vi "initialise.vi"(8 "error in (no error)":errorcluster, 11 "Stimulator090724 in":refnum<class "StimulatorDL090727Writer.lvclass">) -> (0 "error out":errorcluster, 3 "Stimulator090724 out":refnum<class "StimulatorDL090727Writer.lvclass">)   [LabVIEW 2010, in "StimulatorDL090727Writer.lvclass"]
doc: "The dynamic dispatch-version of this VI initalises the plug-in object by allocating and initalising any dynamic resources need."
uses:
  StimulatorDL090727Writer.lvclass
  common/enumerations/functional_global_action_enum.ctl
  StimulatorDL090727Writer.lvclass/StimulatorDL090727Writer.ctl
  SignalWriter/GenericSignalWriter/GenericSignalWriter/GenericSignalWriter.lvclass
  StimulatorDL090724Scaffold/StimulatorDL090724Scaffold/Stimulator090724Scaffold.lvclass
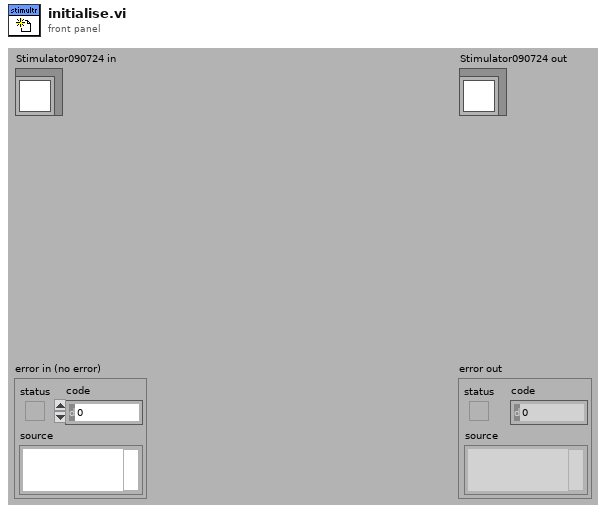
[diagram p1: front panel]
types:
  T1 = typedef "functional_global_action_enum.ctl" = enum16{"get", "set", "reset"}
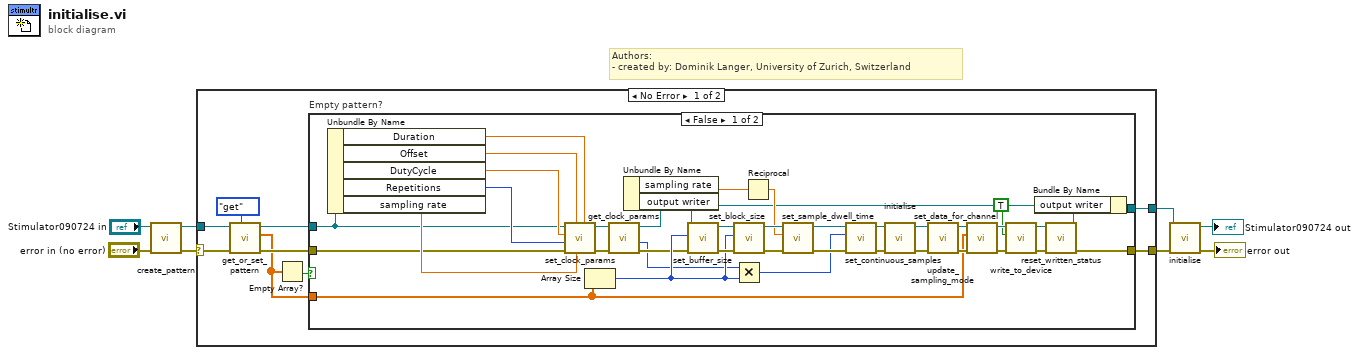
[diagram p0: block diagram]
diagram:
  # "Authors: \n- created by: Dominik Langer, University of Zurich, Switzerland"
  n1 = call-dynamic "create_pattern.vi"("error in (no error)"="error in (no error)", "StimulatorDL090727DAQmx in"="Stimulator090724 in") -> ("error out"=w4:errorcluster, "StimulatorDL090727DAQmx out"=w3:refnum<class "StimulatorDL090727Writer.lvclass">)  [unwired: 8 out]
  n2 = case shown="No Error" w4 {
    selector: w4 -> [w14 w58]
    tunnel: w3 -> [w13 w59]
    tunnel: [w16 w58] -> w2
    tunnel: [w15 w59] -> w1
    frame No Error {
      n3 = call-dynamic "get_or_set_pattern.vi"("action"=functional_global_action_enum."get", "error in (no error)"=w14, "Stimulator090724 in"=w13) -> ("error out"=w12:errorcluster, "samples out"=w10:dbl[], "Stimulator090724 out"=w11:refnum<class "StimulatorDL090727Writer.lvclass">)  [unwired: 1 in, 5 out]
      n4 = Empty Array?(array=w10) -> (empty?=w9:bool)
      n5 = case "Empty pattern?" shown="False" w9 {
        tunnel: w10 -> [w41 _]
        tunnel: [w23 w57] -> w16
        tunnel: [w22 w56] -> w15
        tunnel: w12 -> [w19 w57]
        tunnel: w11 -> [w18 w56]
        frame False {
          n6 = Unbundle By Name(w18) -> ("Duration"=w29:dbl[unit], "Offset"=w33:dbl[unit], "DutyCycle"=w32:dbl[unit], "Repetitions"=w31:i32, "sampling rate"=w30:dbl[unit])
          n7 = call-dynamic "set_clock_params.vi"("duration high"=w29, "frequency"=w30, "offset"=w33, "error in (no error)"=w19, "repetitions"=w31, "duty cycle"=w32, "Stimulator090724Scaffold in"=w18) -> ("error out"=w21:errorcluster, "Stimulator090724Scaffold out"=w20:refnum<class "StimulatorDL090727Writer.lvclass">)  [unwired: 3 in]
          n8 = Array Size(array=w41) -> (size(s)=w39:i32)
          n9 = call-dynamic "get_clock_params.vi"("error in (no error)"=w21, "Stimulator090724Scaffold in"=w20) -> ("error out"=w35:errorcluster, "repetitions"=w34:i32, "Stimulator090724Scaffold out"=w25:refnum<class "StimulatorDL090727Writer.lvclass">)  [unwired: 3 in, 4 out]
          n10 = Unbundle By Name(w25) -> ("sampling rate"=w37:dbl[unit], "output writer"=w28:refnum<class "GenericSignalWriter.lvclass">)
          n11 = call-dynamic "set_buffer_size.vi"("error in (no error)"=w35, "buffer size (samples)"=w39, "GenericWriteSignals.lvclass in"=w28) -> ("error out"=w55:errorcluster, "GenericWriteSignals.lvclass out"=w54:refnum<class "GenericSignalWriter.lvclass">)  [unwired: 7 out]
          n12 = call "set_block_size.vi"("error in (no error)"=w55, "block size (samples)"=w39, "GenericWriteSignals.lvclass in"=w54) -> ("error out"=w53:errorcluster, "GenericWriteSignals.lvclass out"=w52:refnum<class "GenericSignalWriter.lvclass">)  [unwired: 7 in]
          n13 = Multiply(x=w34, y=w39) -> (x*y=w38:i32)
          n14 = Reciprocal(x=w37) -> (1/x=w36:dbl[unit])
          n15 = call-dynamic "set_sample_dwell_time.vi"("error in (no error)"=w53, "sample dwell time"=w36, "GenericWriteSignals.lvclass in"=w52) -> ("error out"=w49:errorcluster, "GenericWriteSignals.lvclass out"=w46:refnum<class "GenericSignalWriter.lvclass">)  [unwired: 7 in]
          n16 = call-dynamic "set_continuous_samples.vi"("error in (no error)"=w49, "continuous samples"=w38, "GenericWriteSignals.lvclass in"=w46) -> ("error out"=w48:errorcluster, "GenericWriteSignals.lvclass out"=w47:refnum<class "GenericSignalWriter.lvclass">)  [unwired: 7 out]
          n17 = call-dynamic "initialise.vi"("error in (no error)"=w48, "GenericPlugin in"=w47) -> ("error out"=w51:errorcluster, "GenericPlugin out"=w50:refnum<class "GenericSignalWriter.lvclass">)  [unwired: 8 out]
          n18 = call-dynamic "update_sampling_mode.vi"("error in (no error)"=w51, "GenericWriteSignals in"=w50) -> ("error out"=w45:errorcluster, "GenericWriteSignals out"=w42:refnum<class "GenericSignalWriter.lvclass">)  [unwired: 8 out]
          n19 = call-dynamic "set_data_for_channel.vi"("error in (no error)"=w45, "data"=w41, "GenericWriteSignals in"=w42) -> ("error out"=w44:errorcluster, "GenericWriteSignals out"=w43:refnum<class "GenericSignalWriter.lvclass">)  [unwired: 7 out]
          n20 = call-dynamic "write_to_device.vi"("error in (no error)"=w44, "force writing?"=TRUE, "GenericWriteSignals in"=w43) -> ("error out"=w27:errorcluster, "GenericWriteSignals out"=w26:refnum<class "GenericSignalWriter.lvclass">)  [unwired: 7 out]
          n21 = call-dynamic "reset_written_status.vi"("error in (no error)"=w27, "GenericWriteSignals in"=w26) -> ("error out"=w23:errorcluster, "GenericWriteSignals out"=w24:refnum<class "GenericSignalWriter.lvclass">)  [unwired: 8 out]
          n22 = Bundle By Name(cluster=w25, "output writer"=w24) -> (w22:refnum<class "StimulatorDL090727Writer.lvclass">)
        }
        frame True {
        }
      }
    }
    frame Error {
    }
  }
  n23 = call-parent "initialise.vi"("error in (no error)"=w2, "Stimulator090724 in"=w1) -> ("error out"=→"error out":errorcluster, "Stimulator090724 out"=→"Stimulator090724 out":refnum<class "StimulatorDL090727Writer.lvclass">)  [unwired: 8 out]
